vi "FFM_actuator_Left.vi"(10 "Force_reference_L":sgl, 11 "V_TF_L":i32) -> (3 "숫자형":i16)   [LabVIEW 2019]
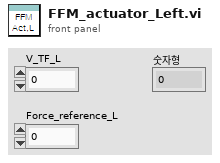
[diagram p1: front panel]
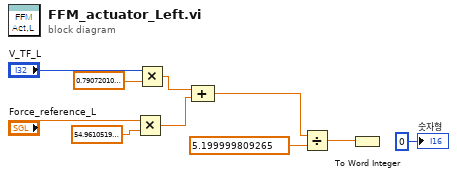
[diagram p0: block diagram]
diagram:
  n1 = Multiply(x="Force_reference_L", y=54.96105194091797) -> (x*y=w6:dbl)
  n2 = Multiply(x="V_TF_L", y=sgl 0.7907201) -> (x*y=w5:sgl)
  n3 = Compound Arithmetic op=ADD ("복합 연산")(w5, w6) -> (w7:dbl)
  n4 = Divide(x=w7, y=5.199999809265) -> (x/y=w9:dbl)
  n5 = To Word Integer(number=w9) -> ()  [unwired: 1 out]
  "숫자형" <- i16 0 ("숫자형")
